vi "Handle.vi"(8 "error in (no error)":errorcluster, 11 "WeatherStation in":refnum<class "WeatherStation.lvclass">) -> (0 "error out":errorcluster, 3 "WeatherStation out":refnum<class "WeatherStation.lvclass">)   [LabVIEW 2018, in "WeatherStation.lvclass"]
uses:
  WeatherStation.lvclass
  WeatherStation.lvclass/WeatherStation.ctl
  Device/Device.lvclass/Device.ctl
  WeatherSensor/WeatherSensor.lvclass
  C:/Users/orlando/Documents/Orlando/SPARC4/Sparc4GUI/Versao ZeroMQ REQ-REP/SPARC4_GUI -v1.0.6 - set suffix automatico para os ACS/Device/Device.lvclass
  Server/Server.lvclass
  Comm/Stream/Stream.lvclass
  Device/Device.lvclass
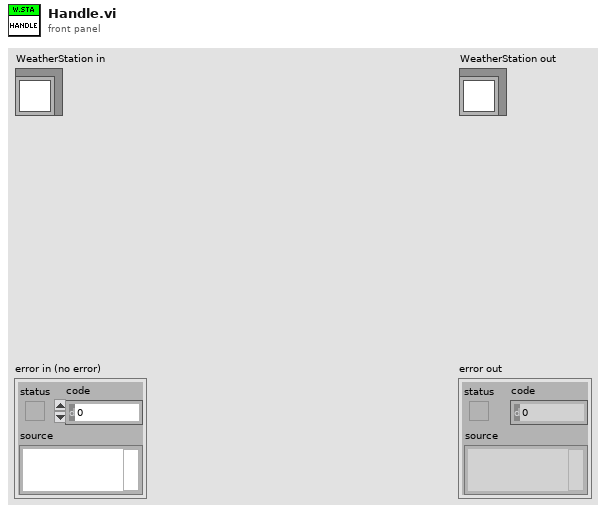
[diagram p1: front panel]
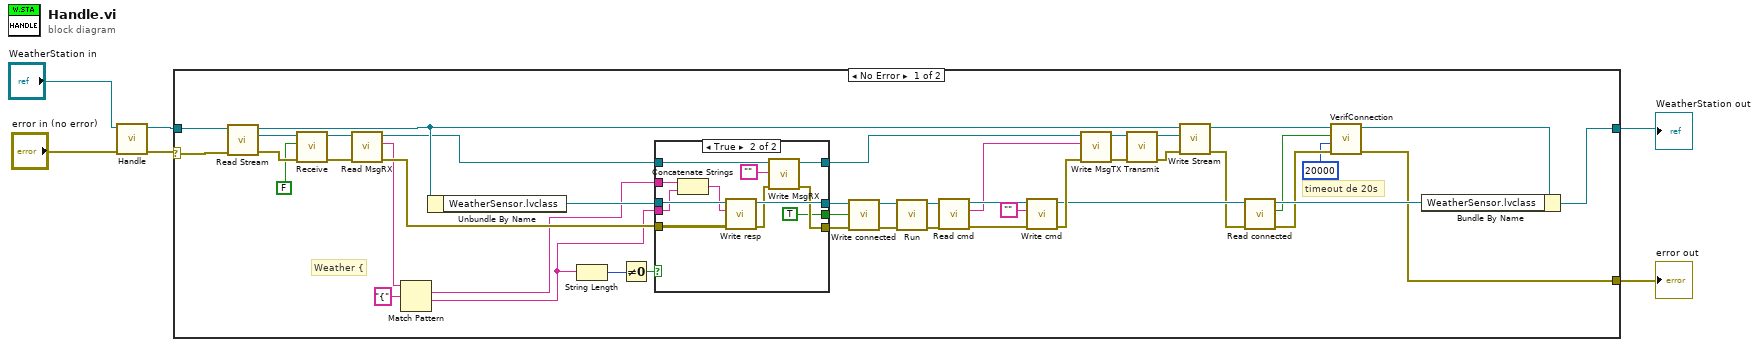
[diagram p0: block diagram]
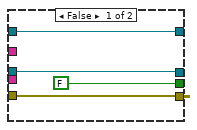
[diagram p2: hidden frame]
diagram:
  n1 = call-parent "Handle.vi"("error in (no error)"="error in (no error)", "Server in"="WeatherStation in") -> ("error out"=w3:errorcluster, "Server out"=w4:refnum<class "WeatherStation.lvclass">)  [unwired: 8 in]
  n2 = case shown="No Error" w3 {
    selector: w3 -> [w48 w68]
    tunnel: [w23 w68] -> w2
    tunnel: [w47 w67] -> w1
    tunnel: w4 -> [w40 w67]
    frame No Error {
      # "Weather {"
      # "timeout de 20s"
      n3 = call-dynamic "Read Stream.vi"("error in (no error)"=w48, "Server in"=w40) -> ("error out"=w49:errorcluster, "Stream.lvclass"=w50:refnum<class "Stream.lvclass">, "Server out"=w21:refnum<class "WeatherStation.lvclass">)  [unwired: 7 in]
      n4 = call-dynamic "Receive.vi"("error in (no error)"=w49, "log?"=FALSE, "Stream in"=w50) -> ("error out"=w46:errorcluster, "Stream out"=w45:refnum<class "Stream.lvclass">)  [unwired: 7 in]
      n5 = call-dynamic "Read MsgRX.vi"("error in (no error)"=w46, "Comm in"=w45) -> ("error out"=w19:errorcluster, "MsgRX"=w11:string, "Comm out"=w14:refnum<class "Stream.lvclass">)  [unwired: 7 in]
      n6 = Match Pattern(string=w11, regular expression="{") -> (match substring=w8:string, after substring=w9:string)  [unwired: 1 in, 2 out]
      n7 = Unbundle By Name(w21) -> ("WeatherSensor.lvclass"=w20:refnum<class "WeatherSensor.lvclass">)
      n8 = String Length(string=w9) -> (length=w34:i32)
      n9 = Not Equal To 0?(x=w34) -> (x != 0?=w33:bool)
      n10 = case shown="True" w33 {
        tunnel: [w53 w60] -> w16
        tunnel: [w54 w65] -> w18
        tunnel: w19 -> [w53 w64]
        tunnel: w20 -> [w54 w66]
        tunnel: w9 -> [_ w56]
        tunnel: w14 -> [w51 w63]
        tunnel: [w51 w62] -> w13
        tunnel: [FALSE TRUE] -> w12
        tunnel: w8 -> [_ w57]
        frame False {
        }
        frame True {
          n11 = Concatenate Strings(w57, w56) -> (w55:string)
          n12 = call-dynamic "Write resp.vi"("error in (no error)"=w64, "resp"=w55, "Device in"=w66) -> ("error out"=w61:errorcluster, "Device out"=w65:refnum<class "WeatherSensor.lvclass">)  [unwired: 7 in]
          n13 = call-dynamic "Write MsgRX.vi"("error in (no error)"=w61, "MsgRX"="", "Comm in"=w63) -> ("error out"=w60:errorcluster, "Comm out"=w62:refnum<class "Stream.lvclass">)  [unwired: 7 in]
        }
      }
      n14 = call "Write connected.vi"("error in (no error)"=w16, "connected"=w12, "Device in"=w18) -> ("error out"=w15:errorcluster, "Device out"=w17:refnum<class "WeatherSensor.lvclass">)  [unwired: 7 in]
      n15 = call-dynamic "Run.vi"("error in (no error)"=w15, "WeatherSensor in"=w17) -> ("error out"=w31:errorcluster, "WeatherSensor out"=w32:refnum<class "WeatherSensor.lvclass">)  [unwired: 8 in]
      n16 = call-dynamic "Read cmd.vi"("error in (no error)"=w31, "Device in"=w32) -> ("error out"=w38:errorcluster, "cmd"=w36:string, "Device out"=w39:refnum<class "WeatherSensor.lvclass">)  [unwired: 7 in]
      n17 = call-dynamic "Write cmd.vi"("error in (no error)"=w38, "cmd"="", "Device in"=w39) -> ("error out"=w44:errorcluster, "Device out"=w30:refnum<class "WeatherSensor.lvclass">)  [unwired: 7 in]
      n18 = call-dynamic "Write MsgTX.vi"("error in (no error)"=w44, "MsgTX"=w36, "Comm in"=w13) -> ("error out"=w42:errorcluster, "Comm out"=w43:refnum<class "Stream.lvclass">)  [unwired: 7 in]
      n19 = call-dynamic "Transmit.vi"("error in (no error)"=w42, "Stream in"=w43) -> ("error out"=w41:errorcluster, "Stream out"=w35:refnum<class "Stream.lvclass">)  [unwired: 8 in]
      n20 = call-dynamic "Write Stream.vi"("error in (no error)"=w41, "Stream.lvclass"=w35, "Server in"=w21) -> ("error out"=w29:errorcluster, "Server out"=w28:refnum<class "WeatherStation.lvclass">)  [unwired: 7 in]
      n21 = call "Read connected.vi"("error in (no error)"=w29, "Device in"=w30) -> ("error out"=w24:errorcluster, "connected"=w26:bool, "Device out"=w27:refnum<class "WeatherSensor.lvclass">)  [unwired: 7 in]
      n22 = call-dynamic "VerifConnection.vi"("error in (no error)"=w24, "timeout in ms (1000)"=u32 20000 ("period (ms)"), "device connected in"=w26, "Server in"=w28) -> ("error out"=w23:errorcluster, "Server out"=w25:refnum<class "WeatherStation.lvclass">)  [unwired: 6 in]
      n23 = Bundle By Name(cluster=w25, "WeatherSensor.lvclass"=w27) -> (w47:refnum<class "WeatherStation.lvclass">)
    }
    frame Error {
    }
  }
  "error out" <- w2
  "WeatherStation out" <- w1
